vi "SER_RAND_V3.vi"() -> ()   [LabVIEW 2018]
uses:
  Var_serrure.vi
  Var_serrure2.vi
panel:
  in  "Combinaison a prendre":i16
  out "Nombre Random":dbl[](array[numeric])
  in  "Nombre d'entier souhaité":i16
  out "i":picture
  out "MAX":dbl
  in  "?":bool
  out "Combinaison":dbl
  out "CURRENT":dbl
  out "Nombre_entrer":dbl
  in  "?":bool
  out "LED ROUGE":bool
  out "LED VERTE":bool
  in  "Nr3":u8(knob) max=9 step=1 scale=0.0..9.0
  in  "Nr2":u8(knob) max=9 step=1 scale=0.0..9.0
  in  "Nr1":u8(knob) max=9 step=1 scale=0.0..9.0
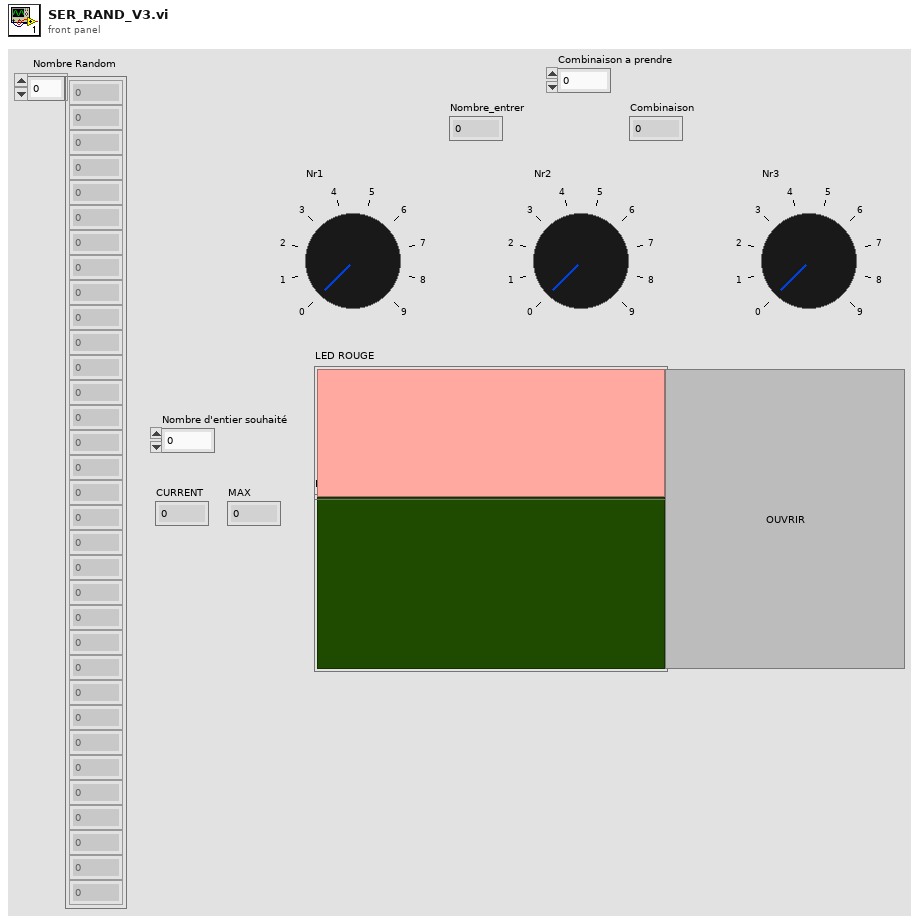
[diagram p1: front panel]
types:
  T1 = typedef "imagedata.ctl" = cluster{"image type":i32, "image depth":i32, "image":u8[], "mask":u8[], "colors":u32[], "Rectangle":cluster{"left":i16, "top":i16, "right":i16, "bottom":i16}}
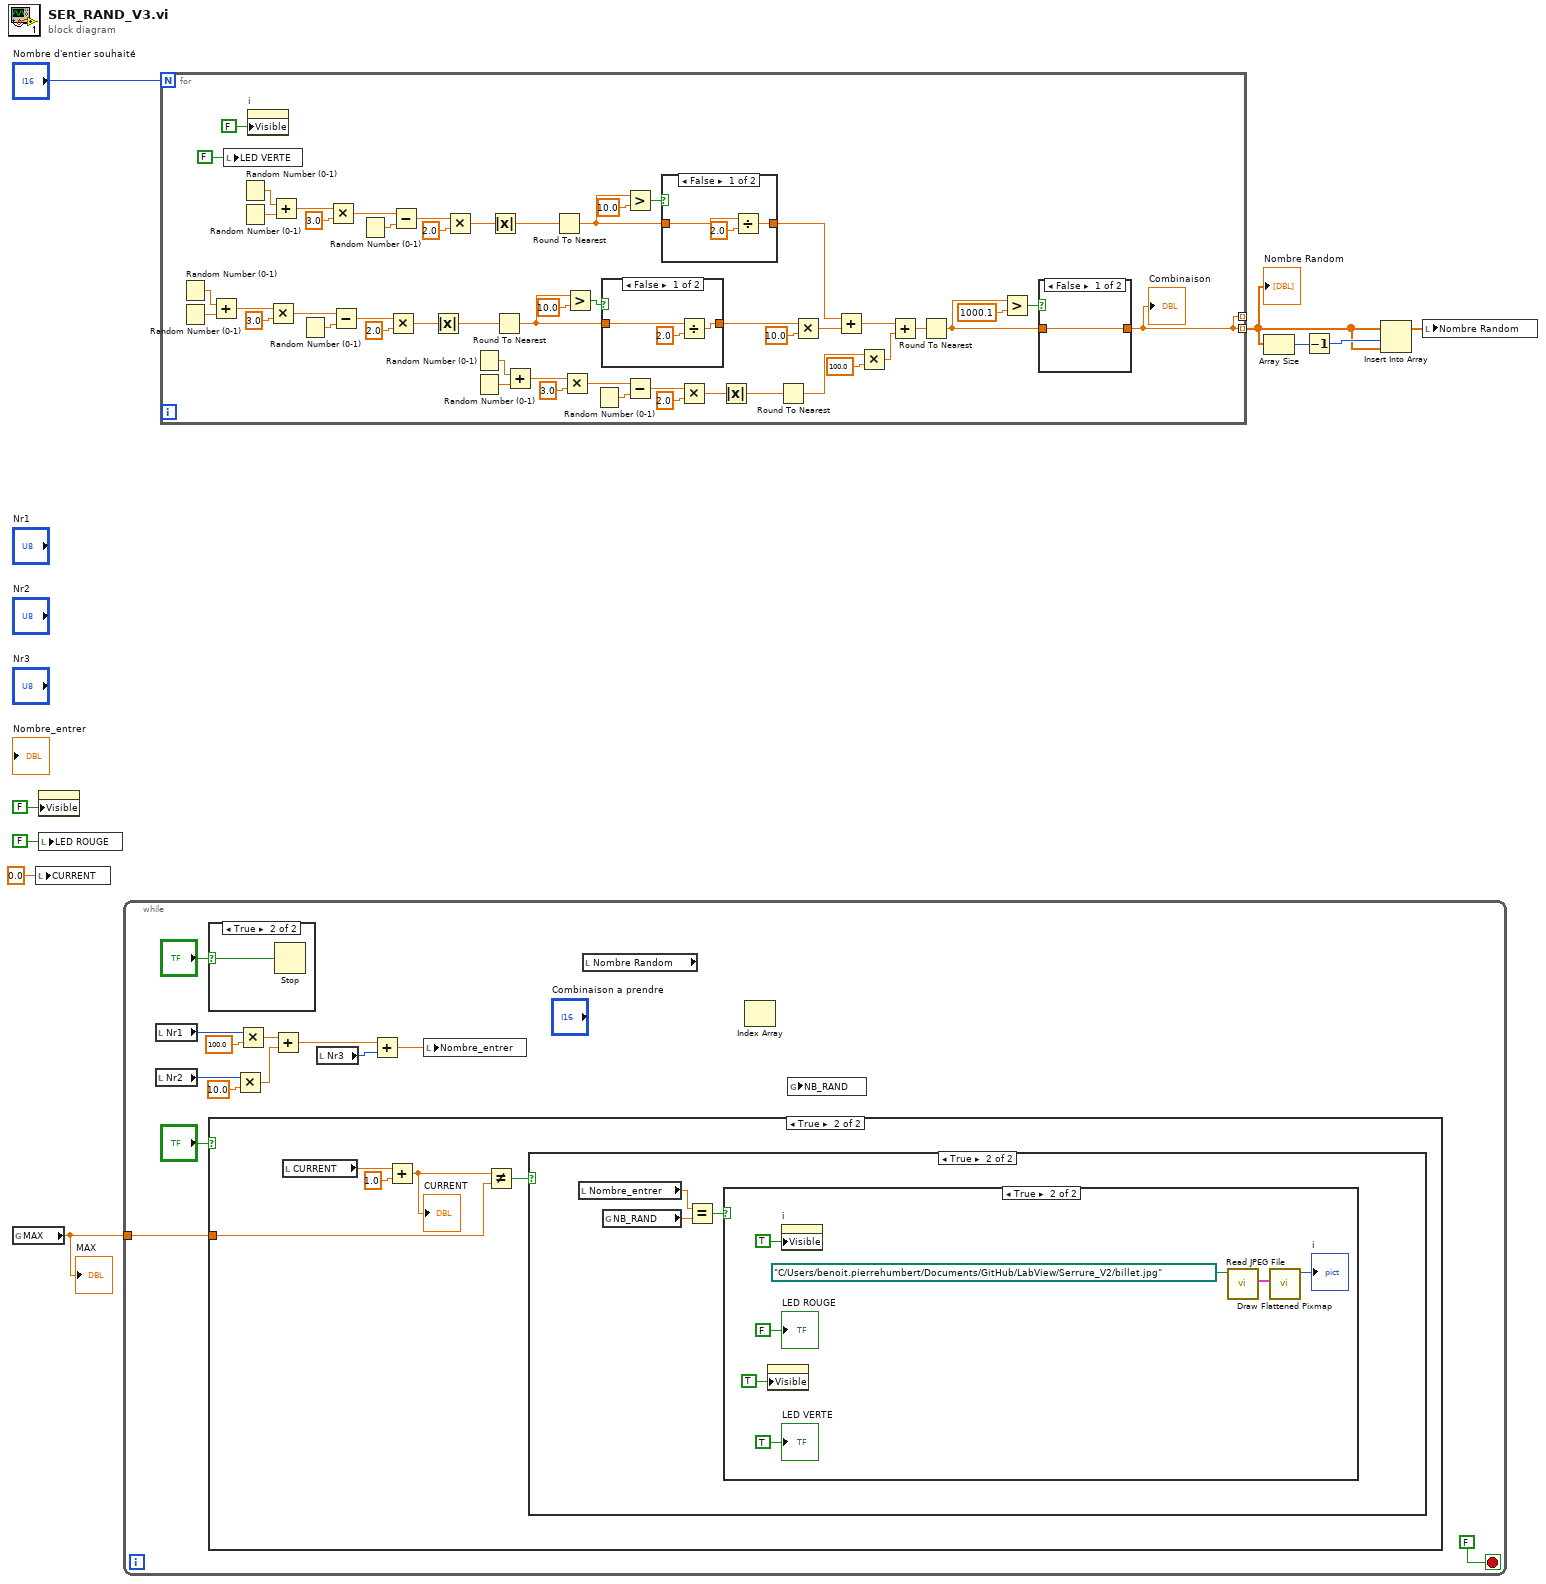
[diagram p0: block diagram]
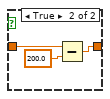
[diagram p2: hidden frame]
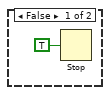
[diagram p7: hidden frame]
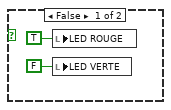
[diagram p8: hidden frame]
diagram:
  n1 = global read "Var_serrure2.vi" "MAX"() -> (w7:dbl)
  "MAX" <- w7
  n2 = local write "CURRENT"(0.0 ("CURRENT")) -> ()
  n3 = property class="Bool"("Visible"=FALSE) -> ()  [unwired: 2 in, 2 out]
  n4 = local write "LED ROUGE"(FALSE ("LED ROUGE")) -> ()
  n5 = while {
    tunnel: w7 -> [w10]
    stop <- FALSE stop-if-true
    n6 = local read "Nr1"() -> (w20:u8)
    n7 = local read "Nr2"() -> (w19:u8)
    n8 = case shown="True" "?" {
      selector: "?" -> [_ w23]
      frame False {
      }
      frame True {
        n9 = Stop(stop? (T)=w23) -> ()
      }
    }
    n10 = case shown="True" "?" {
      tunnel: w10 -> [_ w28]
      frame False {
      }
      frame True {
        n11 = local read "CURRENT"() -> (w27:dbl)
        n12 = Add(x=w27, y=1.0) -> (x+y=w24:dbl)
        "CURRENT" <- w24
        n13 = Not Equal?(x=w24, y=w28) -> (x != y?=w25:bool)
        n14 = case shown="True" w25 {
          frame False {
            n15 = Stop(stop? (T)=TRUE) -> ()
          }
          frame True {
            n16 = local read "Nombre_entrer"() -> (w31:dbl)
            n17 = global read "Var_serrure.vi" "NB_RAND"() -> (w32:ext)
            n18 = Equal?(x=w31, y=w32) -> (x = y?=w30:bool)
            n19 = case shown="True" w30 {
              frame False {
                n20 = local write "LED ROUGE"(TRUE ("LED ROUGE")) -> ()
                n21 = local write "LED VERTE"(FALSE ("LED VERTE")) -> ()
              }
              frame True {
                n22 = property class="Bool"("Visible"=TRUE) -> ()  [unwired: 2 in, 2 out]
                n23 = property on="i" class="Pict"("Visible"=TRUE) -> ()  [unwired: 2 in, 2 out]
                n24 = call <vilib>:"Read JPEG File.vi"("path to JPEG file"=path "C:/Users/benoit.pierrehumbert/Documents/GitHub/LabView/Serrure_V2/billet.jpg") -> ("image data"=w37:T1)  [unwired: 8 in, 2 out]
                n25 = call <vilib>:"Draw Flattened Pixmap.vi"("image data"=w37) -> ("new picture"=→"i":picture)  [unwired: 8 in]
                "LED VERTE" <- TRUE ("LED VERTE")
                "LED ROUGE" <- FALSE ("LED ROUGE")
              }
            }
          }
        }
      }
    }
    n26 = Multiply(x=w19, y=10.0) -> (x*y=w16:dbl)
    n27 = Multiply(x=w20, y=100.0) -> (x*y=w15:dbl)
    n28 = Add(x=w15, y=w16) -> (x+y=w18:dbl)
    n29 = local read "Nr3"() -> (w17:u8)
    n30 = Add(x=w18, y=w17) -> (x+y=w14:dbl)
    n31 = local write "Nombre_entrer"(w14) -> ()
    n32 = local read "Nombre Random"() -> ()  [unwired: 1 out]
    n33 = Index Array() -> ()  [unwired: 2 in, 1 out]
    n34 = global read "Var_serrure.vi" "NB_RAND"() -> ()  [unwired: 1 in]
  }
  n35 = for {
    N: "Nombre d'entier souhaité" -> [_]
    tunnel: [w42] -> w1 mode=indexing
    tunnel: [w42] -> _ mode=indexing
    n36 = Random Number (0-1)() -> (number: 0 to 1=w67:dbl)
    n37 = Random Number (0-1)() -> (number: 0 to 1=w68:dbl)
    n38 = Add(x=w67, y=w68) -> (x+y=w69:dbl)
    n39 = local write "LED VERTE"(FALSE ("LED VERTE")) -> ()
    n40 = Random Number (0-1)() -> (number: 0 to 1=w56:dbl)
    n41 = Random Number (0-1)() -> (number: 0 to 1=w57:dbl)
    n42 = property on="i" class="Pict"("Visible"=FALSE) -> ()  [unwired: 2 in, 2 out]
    n43 = Multiply(x=w69, y=3.0) -> (x*y=w70:dbl)
    n44 = Add(x=w56, y=w57) -> (x+y=w58:dbl)
    n45 = Random Number (0-1)() -> (number: 0 to 1=w71:dbl)
    n46 = Multiply(x=w58, y=3.0) -> (x*y=w59:dbl)
    n47 = Subtract(x=w70, y=w71) -> (x-y=w72:dbl)
    n48 = Random Number (0-1)() -> (number: 0 to 1=w60:dbl)
    n49 = Multiply(x=w72, y=2.0) -> (x*y=w75:dbl)
    n50 = Subtract(x=w59, y=w60) -> (x-y=w61:dbl)
    n51 = Absolute Value(x=w75) -> (abs(x)=w73:dbl)
    n52 = Multiply(x=w61, y=2.0) -> (x*y=w64:dbl)
    n53 = Random Number (0-1)() -> (number: 0 to 1=w77:dbl)
    n54 = Random Number (0-1)() -> (number: 0 to 1=w78:dbl)
    n55 = Absolute Value(x=w64) -> (abs(x)=w62:dbl)
    n56 = Round To Nearest(number=w73) -> (nearest integer value=w76:dbl)
    n57 = Add(x=w77, y=w78) -> (x+y=w79:dbl)
    n58 = Round To Nearest(number=w62) -> (nearest integer value=w65:dbl)
    n59 = Multiply(x=w79, y=3.0) -> (x*y=w80:dbl)
    n60 = Greater?(x=w76, y=10.0) -> (0:w74:bool)
    n61 = Random Number (0-1)() -> (number: 0 to 1=w81:dbl)
    n62 = case shown="False" w74 {
      tunnel: w76 -> [w99 w100]
      tunnel: [w97 w100] -> w85
      frame False {
        n63 = Divide(x=w99, y=2.0) -> (x/y=w97:dbl)
      }
      frame True {
      }
    }
    n64 = Greater?(x=w65, y=10.0) -> (0:w63:bool)
    n65 = Subtract(x=w80, y=w81) -> (x-y=w82:dbl)
    n66 = case shown="False" w63 {
      tunnel: w65 -> [w103 w104]
      tunnel: [w101 w104] -> w66
      frame False {
        n67 = Divide(x=w103, y=2.0) -> (x/y=w101:dbl)
      }
      frame True {
      }
    }
    n68 = Multiply(x=w82, y=2.0) -> (x*y=w84:dbl)
    n69 = Absolute Value(x=w84) -> (abs(x)=w83:dbl)
    n70 = Round To Nearest(number=w83) -> (nearest integer value=w90:dbl)
    n71 = Multiply(x=w85, y=10.0) -> (x*y=w86:dbl)
    n72 = Add(x=w66, y=w86) -> (x+y=w87:dbl)
    n73 = Multiply(x=w90, y=100.0) -> (x*y=w88:dbl)
    n74 = Add(x=w87, y=w88) -> (x+y=w89:dbl)
    n75 = Round To Nearest(number=w89) -> (nearest integer value=w92:dbl)
    n76 = Greater?(x=w92, y=1000.1) -> (0:w91:bool)
    n77 = case shown="False" w91 {
      tunnel: w92 -> [w93 w96]
      tunnel: [w93 w94] -> w42
      frame False {
      }
      frame True {
        n78 = Subtract(x=w96, y=200.0) -> (x-y=w94:dbl)
      }
    }
    "Combinaison" <- w42
  }
  "Nombre Random" <- w1
  n79 = Array Size(array=w1) -> (size(s)=w5:i32)
  n80 = Decrement(x=w5) -> (x-1=w4:i32)
  n81 = Insert Into Array(array=w1, index=w4, new element=w1) -> (w2:dbl[])
  n82 = local write "Nombre Random"(w2) -> ()
